vi "setup.vi"() -> ()   [LabVIEW 2015]
doc: "setup dialog"
panel:
  in  "Tree":string(tree)
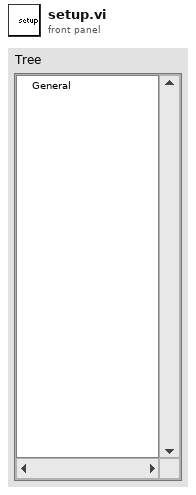
[diagram p1: front panel]
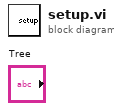
[diagram p0: block diagram]
diagram:
